vi "STOPPED FUNCTION.vi"(8 "Error In Cluster":T3={"Unhandled Error"=FALSE, "Error"={"status"=FALSE, "code"=0, "source"=""}, "Message Type"=enum."Code", "Number of Values"=0, "Msg Value Type"=[], "Msg Ints"=[], "Msg Real Values"=[], "Msg String Values"=[], "Severity (Emergency)"=enum."Emergency"} {"Msg Real Values" format="%.2f"}, 10 "Tags":T1[](array[typedef]), 11 "Source":refnum<class "Source.lvclass">) -> (0 "Error Out Cluster":T2={"Unhandled Error"=FALSE, "Error"={"status"=FALSE, "code"=0, "source"=""}, "Message Type"=enum."Code", "Number of Values"=0, "Msg Value Type"=[], "Msg Ints"=[], "Msg Real Values"=[], "Msg String Values"=[], "Severity (Emergency)"=enum."Emergency"} {"Msg Real Values" format="%.2f"})   [LabVIEW 2013, in "Customer.TestSLATE.Mnemonic.lvlib"]
uses:
  Customer.TestSLATE.Mnemonic.lvlib
  <vilib>/Test SLATE/CONTROLS/Error In Cluster.ctl
  <vilib>/Test SLATE/CONTROLS/Error Out Cluster.ctl
  <vilib>/Test SLATE/CLASSES/SOURCE/Source.lvclass
  <vilib>/Test SLATE/CVT/Tag Information.ctl
  <vilib>/Test SLATE/CLASSES/TAG/TS_Tag.lvclass
  <vilib>/Test SLATE/COMMON/Test Executive Commonl.vi
  <vilib>/Test SLATE/BUF_AI/Write AI Raw to Data Storage Time Stamped.vi
  <vilib>/Test SLATE/BUF_FI/Write FI Raw to Data Storage Time Stamped.vi
  <vilib>/Test SLATE/BUF_CA/Write CA Raw to Data Storage Time Stamped.vi
  <vilib>/Test SLATE/BUF_DI/Write DI Raw to Data Storage Time Stamped.vi
  <vilib>/Test SLATE/BUF_AO/Write AO Raw to Data Storage Time Stamped.vi
  <vilib>/Test SLATE/BUF_CH/Write CH Raw to Data Storage Time Stamped.vi
  <vilib>/Test SLATE/CVT_DO/DO Common Array.vi
  <vilib>/Test SLATE/BUF_DO/Write DO Raw to Data Storage Time Stamped.vi
  <vilib>/Test SLATE/Test SLATE.lvlib
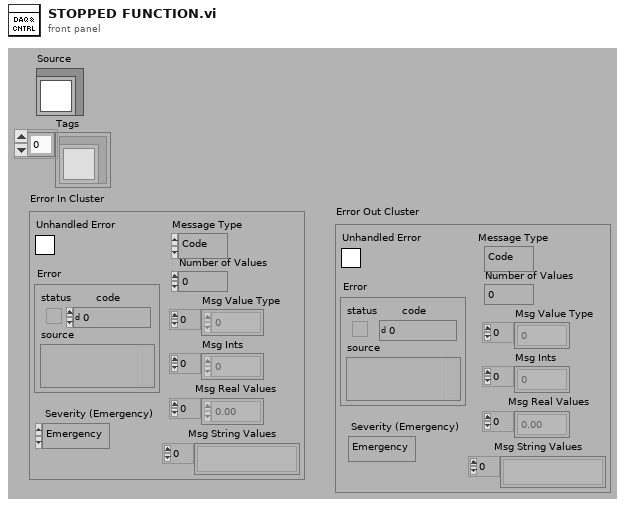
[diagram p1: front panel]
types:
  T1 = typedef "Test SLATE.lvlib/Tag Information.ctl" = refnum<class "TS_Tag.lvclass">
  T2 = typedef "Test SLATE.lvlib/Error Out Cluster.ctl" = cluster{"Unhandled Error":bool, "Error":errorcluster, "Message Type":enum8{"Code", "Text"}, "Number of Values":i8, "Msg Value Type":i32[], "Msg Ints":i32[], "Msg Real Values":sgl[], "Msg String Values":string[], "Severity (Emergency)":enum32{"Information", "Warning", "Emergency"}}
  T3 = typedef "Test SLATE.lvlib/Error In Cluster.ctl" = cluster{"Unhandled Error":bool, "Error":errorcluster, "Message Type":enum8{"Code", "Text"}, "Number of Values":i8, "Msg Value Type":i32[], "Msg Ints":i32[], "Msg Real Values":sgl[], "Msg String Values":string[], "Severity (Emergency)":enum32{"Information", "Warning", "Emergency"}}
  T4 = cluster{"Last Error":i32, "Error Active":bool, "AI Chan Status":i32[], "FI Chan Status":i32[], "CA Chan Status":i32[], "AO Chan Status":i32[], "DI Chan Status":i32[], "DO Chan Status":i32[], "CH Chan Status":i32[]}
  T5 = cluster{"DateOffset":i32, "TimeOffset":i32, "MsecsOffset":i32}
  T6 = cluster{"AI Tag Offset":i32, "FI Tag Offset":i32, "DI Tag Offset":i32, "AO Tag Offset":i32, "DO Tag Offset":i32, "CA Tag Offset":i32, "CH Tag Offset":i32}
  T7 = cluster{"AI Tag Count":i16, "FI Tag Count":i16, "DI Tag Count":i16, "AO Tag Count":i16, "DO Tag Count":i16, "CA Tag Count":i16, "CH Tag Count":i16}
  T8 = typedef "Customer.TestSLATE.Mnemonic.lvlib/Source Status Information.ctl" = cluster{"Indexes":i32[], "Names":string[], "Bad Codes":bool[], "Low Ranges":sgl[], "High Ranges":sgl[]}
  T9 = enum16{"Started", "Stopped", "Initializing", "Acquiring", "Calibrating", "Diagnostics", "Inactive"}
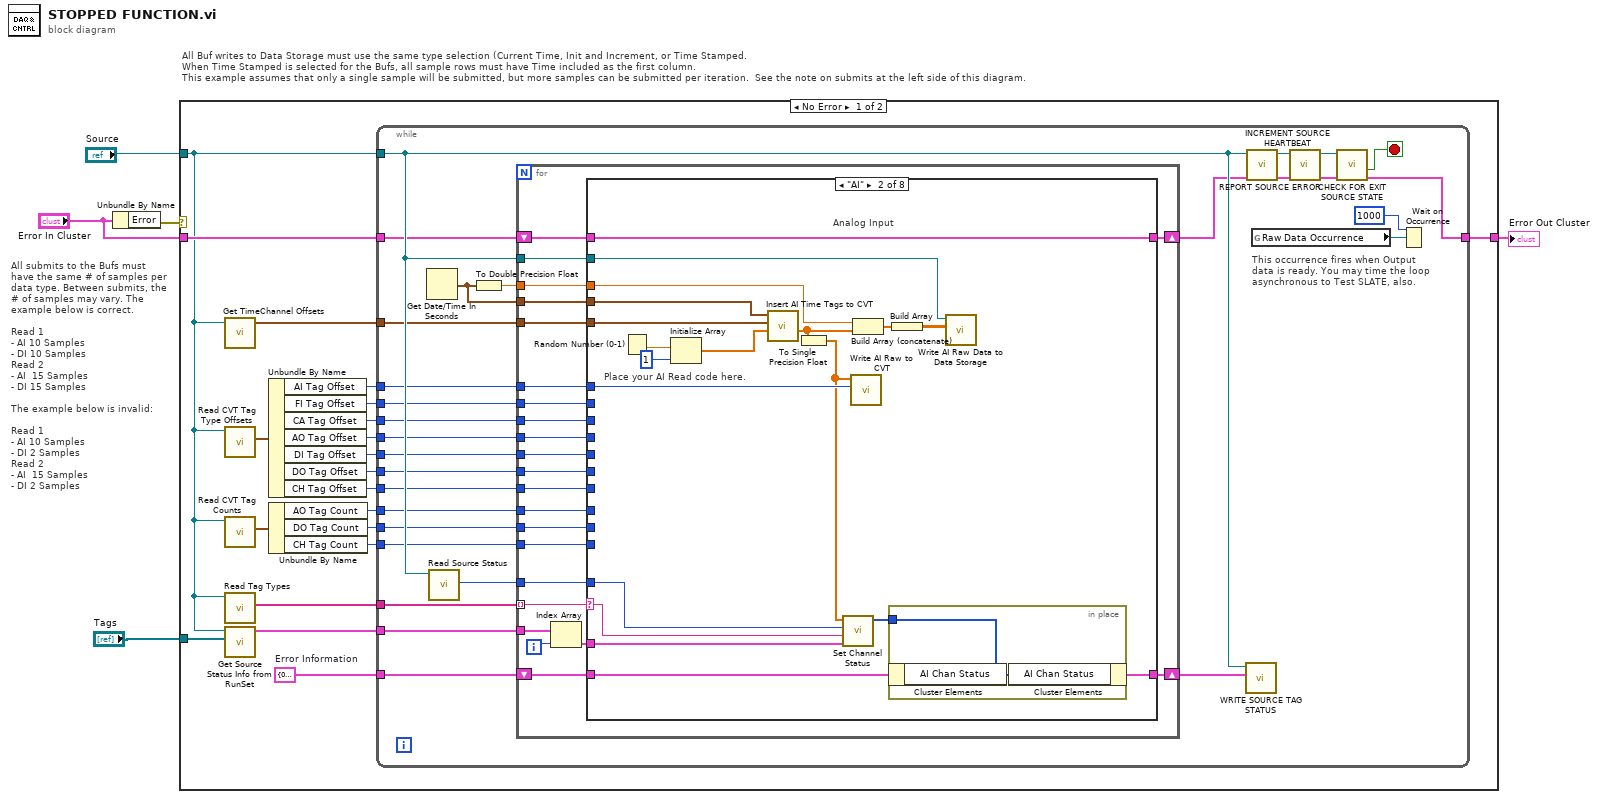
[diagram p0: block diagram]
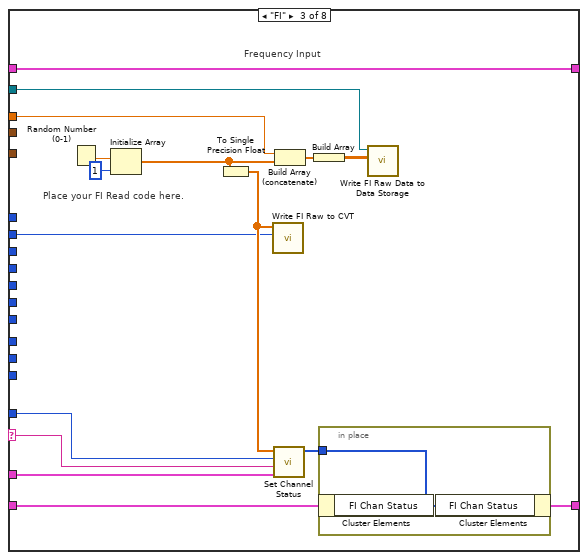
[diagram p3: hidden frame]
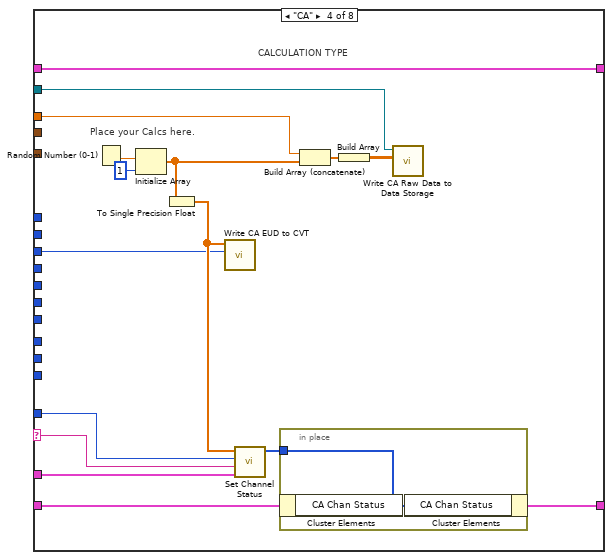
[diagram p4: hidden frame]
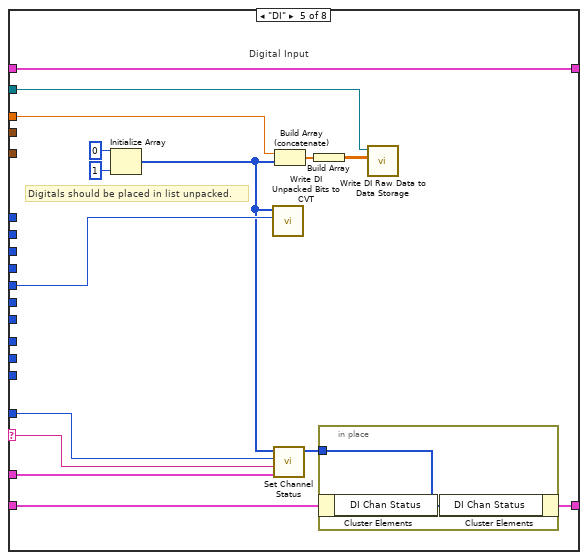
[diagram p5: hidden frame]
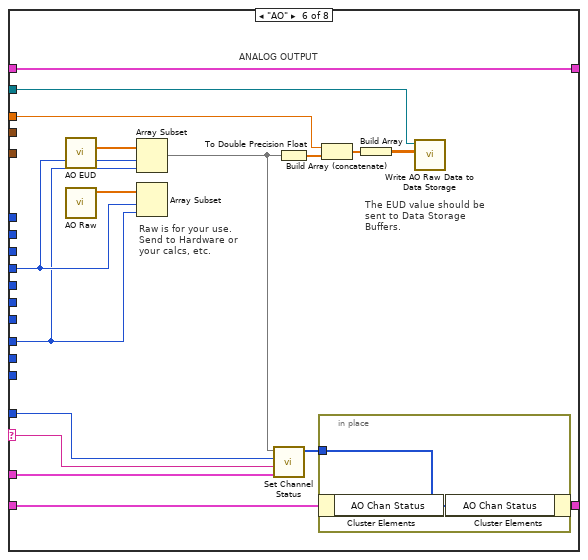
[diagram p6: hidden frame]
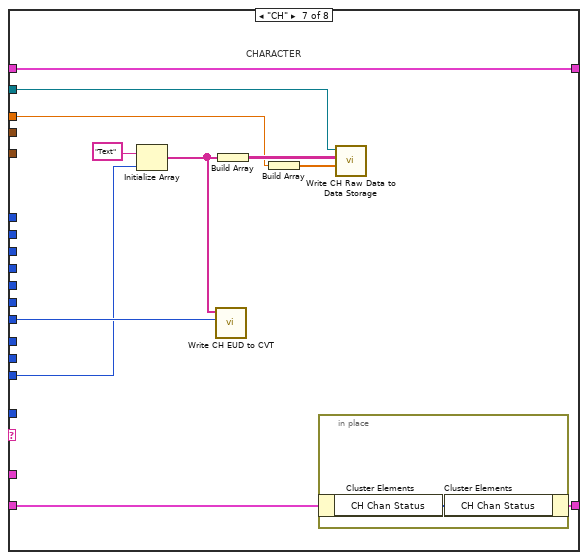
[diagram p7: hidden frame]
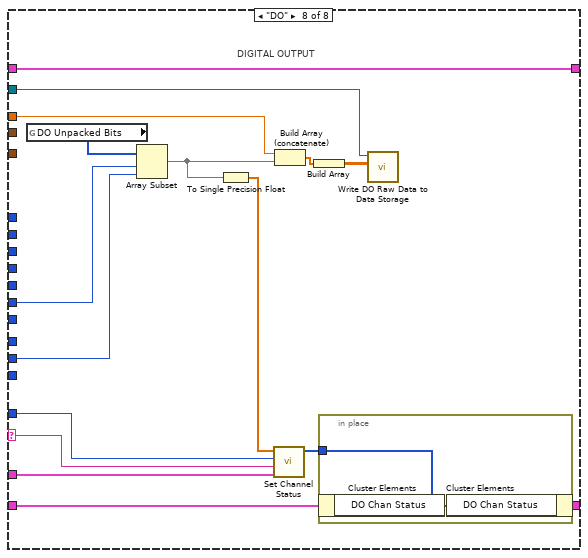
[diagram p8: hidden frame]
diagram:
  # "All Buf writes to Data Storage must use the same type selection (Current Time, Init and Increment, or Time Stamped.\nWhen Time Stamped is selected for the Bufs, all sample rows must have Time included as the first column.\nThis example assumes that only a single sample will be submitted, but more samples can be submitted per iteration.  See the note on submits at the left side of this diagram."
  # "All submits to the Bufs must have the same # of samples per data type. Between submits, the # of samples may vary. The example below is correct.\n\nRead 1 \n- AI 10 Samples\n- DI 10 Samples\nRead 2 \n- AI  15 Samples\n- DI 15 Samples\n\nThe example below is invalid:\n\nRead 1 \n- AI 10 Samples\n- DI 2 Samples\nRead 2 \n- AI  15 Samples\n- DI 2 Samples"
  n1 = Unbundle By Name("Error In Cluster") -> ("Error"=w5:errorcluster)
  n2 = case shown="No Error" w5 {
    tunnel: [w24 w197] -> w3
    tunnel: "Error In Cluster" -> [w25 w197]
    tunnel: "Source" -> [w7 _]
    tunnel: "Tags" -> [w20 _]
    frame No Error {
      w17 = T4 {"Last Error"=0, "Error Active"=FALSE, "AI Chan Status"=[], "FI Chan Status"=[], "CA Chan Status"=[], "AO Chan Status"=[], "DI Chan Status"=[], "DO Chan Status"=[], "CH Chan Status"=[]}  # Error Information
      n3 = call <vilib>:"Get TimeChannel Offsets.vi"("Source"=w7) -> ("Offsets"=w23:T5)  [unwired: 4 in]
      n4 = call <vilib>:"Read CVT Tag Type Offsets.vi"("Source in"=w7) -> ("CVT Tag Offsets"=w22:T6)  [unwired: 9 in, 1 out]
      n5 = call <vilib>:"Read CVT Tag Counts.vi"("Source in"=w7) -> ("Tag Counts"=w10:T7)  [unwired: 9 in, 1 out]
      n6 = call <vilib>:"Read Tag Types.vi"("Source in"=w7) -> ("Tag Types"=w18:string[])  [unwired: 9 in, 1 out]
      n7 = call "Get Source Status Info from RunSet.vi"("Tags"=w20, "Source"=w7) -> ("Tag Status Info"=w19:T8[])  [unwired: 9 in]
      n8 = Unbundle By Name(w22) -> ("AI Tag Offset"=w21:i32, "FI Tag Offset"=w16:i32, "CA Tag Offset"=w15:i32, "AO Tag Offset"=w14:i32, "DI Tag Offset"=w13:i32, "DO Tag Offset"=w12:i32, "CH Tag Offset"=w11:i32)
      n9 = Unbundle By Name(w10) -> ("AO Tag Count"=w9:i16, "DO Tag Count"=w8:i16, "CH Tag Count"=w6:i16)
      n10 = while {
        tunnel: w25 -> [w35]
        tunnel: [w29] -> w24
        tunnel: w23 -> [w50]
        tunnel: w21 -> [w49]
        tunnel: w7 -> [w54]
        tunnel: w19 -> [w47]
        tunnel: w18 -> [w48]
        tunnel: w17 -> [w46]
        tunnel: w16 -> [w43]
        tunnel: w15 -> [w42]
        tunnel: w14 -> [w41]
        tunnel: w13 -> [w40]
        tunnel: w12 -> [w39]
        tunnel: w11 -> [w38]
        tunnel: w9 -> [w37]
        tunnel: w8 -> [w36]
        tunnel: w6 -> [w26]
        stop <- w53 stop-if-true
        # "This occurrence fires when Output\ndata is ready. You may time the loop asynchronous to Test SLATE, also."
        n11 = Get Date/Time In Seconds() -> (seconds since 1Jan1904=w44:timestamp)
        n12 = call <vilib>:"Read Source Status.vi"("Source in"=w54) -> ("Source Status"=w34:T9)  [unwired: 9 in, 1 out]
        n13 = To Double Precision Float(number=w44) -> (double precision float=w45:dbl)
        n14 = for {
          tunnel: w50 -> [w77]
          tunnel: w49 -> [w65]
          tunnel: w54 -> [w76]
          tunnel: w48 -> [w75] mode=indexing
          tunnel: w47 -> [w74]
          shift-right: [w69] -> w27
          shift-left: w46 -> [w71]
          tunnel: w34 -> [w70]
          tunnel: w45 -> [w68]
          tunnel: w44 -> [w67]
          tunnel: w43 -> [w66]
          tunnel: w42 -> [w64]
          tunnel: w41 -> [w63]
          tunnel: w40 -> [w62]
          tunnel: w39 -> [w61]
          tunnel: w38 -> [w60]
          tunnel: w37 -> [w59]
          tunnel: w36 -> [w58]
          shift-right: [w56] -> w33
          shift-left: w35 -> [w57]
          tunnel: w26 -> [w55]
          i -> [w73]
          n15 = Index Array(array=w74, index=w73) -> (element=w72:T8)
          n16 = case shown="\"AI\"" w75 {
            selector: w75 -> [_ w87 w108 w125 w143 w162 _ w190]
            tunnel: w77 -> [_ w98 _ _ _ _ _ _]
            tunnel: w65 -> [_ w97 _ _ _ _ _ _]
            tunnel: w76 -> [_ w96 w115 w132 w148 w166 w178 w195]
            tunnel: w72 -> [_ w88 w109 w126 w144 w163 _ w191]
            tunnel: w71 -> [w79 w84 w105 w122 w140 w159 w177 w187]
            tunnel: w70 -> [_ w85 w106 w123 w141 w160 _ w188]
            tunnel: [w79 w83 w104 w121 w139 w158 w176 w186] -> w69
            tunnel: w68 -> [_ w82 w103 w120 w138 w157 w173 w185]
            tunnel: w67 -> [_ w81 _ _ _ _ _ _]
            tunnel: w66 -> [_ _ w101 _ _ _ _ _]
            tunnel: w64 -> [_ _ _ w118 _ _ _ _]
            tunnel: w63 -> [_ _ _ _ _ w153 _ _]
            tunnel: w62 -> [_ _ _ _ w137 _ _ _]
            tunnel: w61 -> [_ _ _ _ _ _ _ w182]
            tunnel: w60 -> [_ _ _ _ _ _ w170 _]
            tunnel: w59 -> [_ _ _ _ _ w152 _ _]
            tunnel: w58 -> [_ _ _ _ _ _ _ w181]
            tunnel: [w78 w80 w100 w117 w134 w156 w175 w180] -> w56
            tunnel: w57 -> [w78 w80 w100 w117 w134 w156 w175 w180]
            tunnel: w55 -> [_ _ _ _ _ _ w168 _]
            frame "", Default {
            }
            frame "AI" {
              # "Place your AI Read code here."
              # "Analog Input"
              n17 = Random Number (0-1)() -> (number: 0 to 1=w93:dbl)
              n18 = Initialize Array(w93, 1 ("dimension size")) -> (w94:dbl[])
              n19 = call <vilib>:"Insert AI Time Tags to CVT.vi"("AI Input Array"=w94, "Offsets"=w98, "Time"=w81) -> ("AI Output Array"=w95:dbl[])  [unwired: 7 in]
              n20 = To Single Precision Float(number=w95) -> (single precision float=w89:sgl[])
              n21 = call "Set Channel Status.vi"("Status Info"=w88, "Data Type"=w87, "My System Status"=w85, "Real Data"=w89) -> ("Channel Statuses"=w86:u32[])  [unwired: 7 in]
              n22 = call <vilib>:"Write AI Raw to CVT.vi"("Start Type Index"=w97, "AI Raw"=w89) -> ()  [unwired: 10 in]
              n23 = Build Array (concatenate)(w82, w95) -> (w92:dbl[])
              n24 = in-place {
                in-place-border: w86 -> [w99]
                n25 = in-place-cluster #1(w84) -> ()  [unwired: 1 out]
                n26 = in-place-cluster #1("AI Chan Status"=w99) -> (w83:T4)
              }
              n27 = Build Array(w92) -> (w90:dbl[][])
              n28 = call-poly <vilib>:"Write AI Raw Data to Data Storage.vi"("Analog Input Data"=w90, "Source"=w96) -> ()  [unwired: 10 in]
            }
            frame "FI" {
              # "Place your FI Read code here."
              # "Frequency Input"
              n29 = Random Number (0-1)() -> (number: 0 to 1=w114:dbl)
              n30 = Initialize Array(w114, 1 ("dimension size")) -> (w102:dbl[])
              n31 = To Single Precision Float(number=w102) -> (single precision float=w110:sgl[])
              n32 = call <vilib>:"Write FI Raw to CVT.vi"("Start Type Index"=w101, "FI Raw"=w110) -> ()  [unwired: 10 in]
              n33 = call "Set Channel Status.vi"("Status Info"=w109, "Data Type"=w108, "My System Status"=w106, "Real Data"=w110) -> ("Channel Statuses"=w107:u32[])  [unwired: 7 in]
              n34 = Build Array (concatenate)(w103, w102) -> (w113:dbl[])
              n35 = Build Array(w113) -> (w111:dbl[][])
              n36 = in-place {
                in-place-border: w107 -> [w116]
                n37 = in-place-cluster #2(w105) -> ()  [unwired: 1 out]
                n38 = in-place-cluster #2("FI Chan Status"=w116) -> (w104:T4)
              }
              n39 = call-poly <vilib>:"Write FI Raw Data to Data Storage.vi"("Frequency Input Data"=w111, "Source"=w115) -> ()  [unwired: 10 in]
            }
            frame "CA" {
              # "Place your Calcs here."
              # "CALCULATION TYPE"
              n40 = Random Number (0-1)() -> (number: 0 to 1=w131:dbl)
              n41 = Initialize Array(w131, 1 ("dimension size")) -> (w119:dbl[])
              n42 = To Single Precision Float(number=w119) -> (single precision float=w127:sgl[])
              n43 = call <vilib>:"Write CA EUD to CVT.vi"("Start Type Index"=w118, "CA CAL EUD"=w127) -> ()  [unwired: 10 in]
              n44 = call "Set Channel Status.vi"("Status Info"=w126, "Data Type"=w125, "My System Status"=w123, "Real Data"=w127) -> ("Channel Statuses"=w124:u32[])  [unwired: 7 in]
              n45 = in-place {
                in-place-border: w124 -> [w133]
                n46 = in-place-cluster #3(w122) -> ()  [unwired: 1 out]
                n47 = in-place-cluster #3("CA Chan Status"=w133) -> (w121:T4)
              }
              n48 = Build Array (concatenate)(w120, w119) -> (w130:dbl[])
              n49 = Build Array(w130) -> (w128:dbl[][])
              n50 = call-poly <vilib>:"Write CA Raw Data to Data Storage.vi"("Calculated Input Data"=w128, "Source"=w132) -> ()  [unwired: 10 in]
            }
            frame "DI" {
              # "Digitals should be placed in list unpacked."
              # "Digital Input"
              n51 = Initialize Array(u32 0 ("element"), 1 ("dimension size")) -> (w135:u32[])
              n52 = call <vilib>:"Write DI Unpacked Bits to CVT.vi"("Start Type Index"=w137, "DI EUD"=w135) -> ()  [unwired: 10 in]
              n53 = call "Set Channel Status.vi"("Status Info"=w144, "Data Type"=w143, "My System Status"=w141, "Real Data"=w135) -> ("Channel Statuses"=w142:u32[])  [unwired: 7 in]
              n54 = Build Array (concatenate)(w138, w135) -> (w147:dbl[])
              n55 = Build Array(w147) -> (w145:dbl[][])
              n56 = in-place {
                in-place-border: w142 -> [w149]
                n57 = in-place-cluster #4(w140) -> ()  [unwired: 1 out]
                n58 = in-place-cluster #4("DI Chan Status"=w149) -> (w139:T4)
              }
              n59 = call-poly <vilib>:"Write DI Raw Data to Data Storage.vi"("Digital Input Data"=w145, "Source"=w148) -> ()  [unwired: 10 in]
            }
            frame "AO" {
              # "The EUD value should be sent to Data Storage Buffers."
              # "Raw is for your use. Send to Hardware or your calcs, etc."
              # "ANALOG OUTPUT"
              n60 = call <vilib>:"AO EUD.vi"() -> ("AO EUD"=w155:sgl[])  [unwired: 3 in]
              n61 = call <vilib>:"AO Raw.vi"() -> ("AO Raw"=w154:sgl[])  [unwired: 11 in]
              n62 = Array Subset(array=w155, index=w153, length=w152) -> (w151:sgl[])
              n63 = Array Subset(array=w154, index=w153, length=w152) -> ()  [unwired: 1 out]
              n64 = call "Set Channel Status.vi"("Status Info"=w163, "Data Type"=w162, "My System Status"=w160, "Real Data"=w151) -> ("Channel Statuses"=w161:u32[])  [unwired: 7 in]
              n65 = To Double Precision Float(number=w151) -> (double precision float=w150:dbl[])
              n66 = in-place {
                in-place-border: w161 -> [w167]
                n67 = in-place-cluster #5(w159) -> ()  [unwired: 1 out]
                n68 = in-place-cluster #5("AO Chan Status"=w167) -> (w158:T4)
              }
              n69 = Build Array (concatenate)(w157, w150) -> (w165:dbl[])
              n70 = Build Array(w165) -> (w164:dbl[][])
              n71 = call-poly <vilib>:"Write AO Raw Data to Data Storage.vi"("Analog Output Data"=w164, "Source"=w166) -> ()  [unwired: 10 in]
            }
            frame "CH" {
              # "CHARACTER"
              n72 = Initialize Array("Text", w168) -> (w171:string[])
              n73 = call <vilib>:"Write CH EUD to CVT.vi"("Start Type Index"=w170, "CH Text"=w171) -> ()  [unwired: 10 in]
              n74 = Build Array(w171) -> (w174:string[][])
              n75 = Build Array(w173) -> (w172:dbl[])
              n76 = in-place {
                n77 = in-place-cluster #6(w177) -> ("CH Chan Status"=w179:i32[])
                n78 = in-place-cluster #6("CH Chan Status"=w179) -> (w176:T4)
              }
              n79 = call-poly <vilib>:"Write CH Raw Data to Data Storage.vi"("Time Data"=w172, "Character Data"=w174, "Source"=w178) -> ()  [unwired: 9 in]
            }
            frame "DO" {
              # "DIGITAL OUTPUT"
              n80 = global read "DO Common Array.vi" "DO Unpacked Bits"() -> (w184:i16[])
              n81 = Array Subset(array=w184, index=w182, length=w181) -> (w183:i16[])
              n82 = To Single Precision Float(number=w183) -> (single precision float=w192:sgl[])
              n83 = call "Set Channel Status.vi"("Status Info"=w191, "Data Type"=w190, "My System Status"=w188, "Real Data"=w192) -> ("Channel Statuses"=w189:u32[])  [unwired: 7 in]
              n84 = Build Array (concatenate)(w185, w183) -> (w194:dbl[])
              n85 = Build Array(w194) -> (w193:dbl[][])
              n86 = in-place {
                in-place-border: w189 -> [w196]
                n87 = in-place-cluster #7(w187) -> ()  [unwired: 1 out]
                n88 = in-place-cluster #7("DO Chan Status"=w196) -> (w186:T4)
              }
              n89 = call-poly <vilib>:"Write DO Raw Data to Data Storage.vi"("Digital Output Data"=w193, "Source"=w195) -> ()  [unwired: 10 in]
            }
          }
        }
        n90 = call <vilib>:"WRITE SOURCE TAG STATUS.vi"("Error Information"=w27, "Source"=w54) -> ()  [unwired: 8 in, 2 out]
        n91 = call <vilib>:"INCREMENT SOURCE HEARTBEAT.vi"("Error In Cluster"=w33, "Source"=w54) -> ("Error Out Cluster"=w31:T2, "Source out"=w32:refnum<class "Source.lvclass">)  [unwired: 8 in]
        n92 = global read "Test Executive Commonl.vi" "Raw Data Occurrence"() -> (w52:refnum<k4>)
        n93 = call <vilib>:"REPORT SOURCE ERROR.vi"("Error In Cluster"=w31, "Source"=w32) -> ("Error Out Cluster"=w30:T2, "Source Out"=w28:refnum<class "Source.lvclass">)  [unwired: 8 in]
        n94 = call <vilib>:"CHECK FOR EXIT SOURCE STATE.vi"("Error In Cluster"=w30, "Source"=w28) -> ("Error Out Cluster"=w29:T2, "Exit Source State"=w53:bool)  [unwired: 7 in, 1 out]
        n95 = Wait on Occurrence(2:w52, 3:1000 ("ms timeout (-1)")) -> ()  [unwired: 1 in, 1 out]
      }
    }
    frame Error {
    }
  }
  "Error Out Cluster" <- w3
